vi "Boiler Controller.vi"(8 "error in":errorcluster, 11 "Message Queues":T1) -> (0 "error out":errorcluster)   [LabVIEW 2015]
uses:
  support/Message Queue/All Message Queues.ctl
  support/Message Queue/Message Cluster.ctl
  support/Message Queue/Message Queue.lvlib
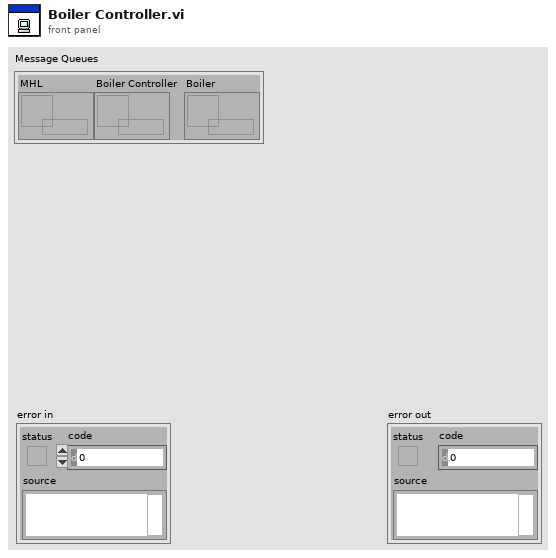
[diagram p1: front panel]
types:
  T1 = typedef "Message Queue.lvlib/All Message Queues.ctl" = cluster{"MHL":refnum<queue>, "Boiler Controller":refnum<queue>, "Boiler":refnum<queue>}
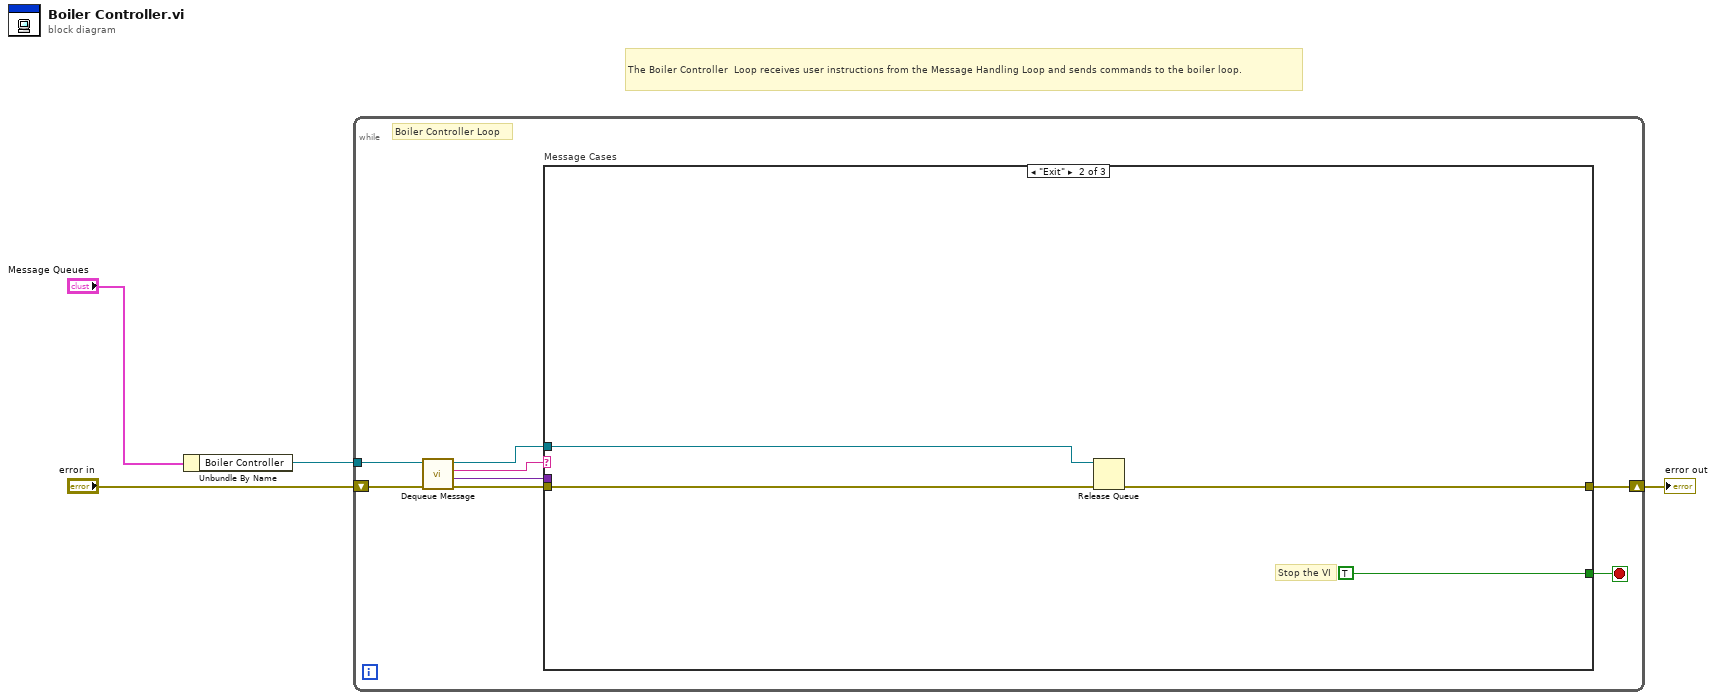
[diagram p0: block diagram]
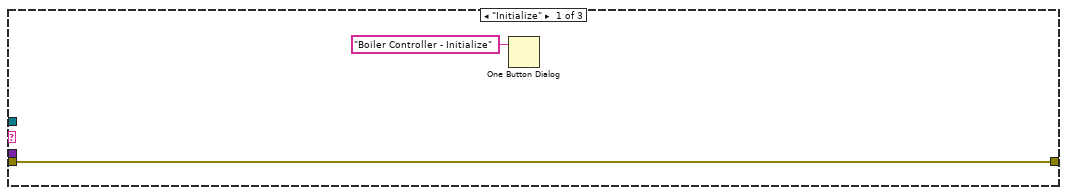
[diagram p2: hidden frame]
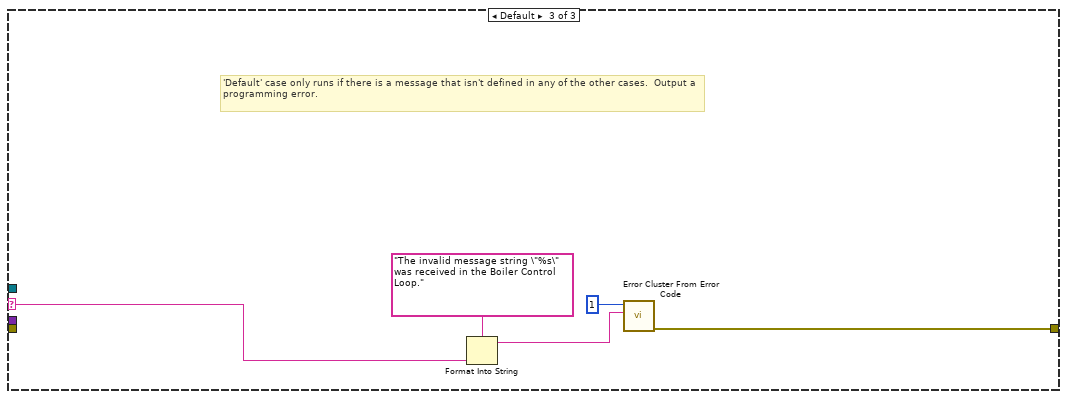
[diagram p3: hidden frame]
diagram:
  # "The Boiler Controller  Loop receives user instructions from the Message Handling Loop and sends commands to the boiler loop."
  n1 = Unbundle By Name("Message Queues") -> ("Boiler Controller"=w2:refnum<queue>)
  n2 = while {
    tunnel: w2 -> [w6]
    shift-right: [w5] -> w4
    shift-left: "error in" -> [w11]
    stop <- w12 stop-if-true
    # "Boiler Controller Loop"
    n3 = call "Dequeue Message.vi"("error in (no error)"=w11, "Message Queue"=w6) -> ("error out"=w10:errorcluster, "Message Data"=w8:variant, "Message"=w9:string, "dup Message Queue"=w7:refnum<queue>)  [unwired: 6 in]
    n4 = case "Message Cases" shown="\"Exit\"" w9 {
      selector: w9 -> [_ _ w20]
      tunnel: w7 -> [_ w17 _]
      tunnel: w10 -> [w14 w16 _]
      tunnel: [w14 w15 w19] -> w5
      tunnel: [_ TRUE _] -> w12
      tunnel: w8 -> [_ _ _]
      frame "Initialize" {
        n5 = One Button Dialog(message="Boiler Controller - Initialize") -> ()  [unwired: 1 in, 1 out]
      }
      frame "Exit" {
        # "Stop the VI"
        n6 = Release Queue(queue=w17, error in (no error)=w16) -> (error out=w15:errorcluster)  [unwired: 1 in, 2 out]
      }
      frame Default {
        # "'Default' case only runs if there is a message that isn't defined in any of the other cases.  Output a programming error."
        n7 = Format Into String(format string="The invalid message string \"%s\" was received in the Boiler Control Loop." ("Unknown Message Error Text"), w20) -> (resulting string=w21:string)  [unwired: 2 in, 1 out]
        n8 = call <vilib>:"Error Cluster From Error Code.vi"("error message (\"\")"=w21, "error code (0)"=1) -> ("error out"=w19:errorcluster)  [unwired: 7 in]
      }
    }
  }
  "error out" <- w4
